vi "Motr_Ref_Num.vi"() -> (0 "Motor":T1)   [LabVIEW 2015]
uses:
  Motor_Type_Def.ctl
  <vilib>/Rock Robotics/WPI/RobotDrive/WPI_RobotDriveDevRef.ctl
  <vilib>/Rock Robotics/WPI/MotorControl/WPI_MotorControlDeviceRef.ctl
  <vilib>/Rock Robotics/WPI/MotorControl/WPI_MotorControlType.ctl
  <vilib>/Rock Robotics/SystemInterfaces/DIO/FPGA_DIOPWMChannel.ctl
  <vilib>/Rock Robotics/WPI/PWM/WPI_PWMDeadband.ctl
  <vilib>/Rock Robotics/WPI/CAN/Jaguar/SubVIs/WPI_CANJaguar_ControlMode.ctl
  <vilib>/Rock Robotics/WPI/CAN/TalonSRX/WPI_CANTalonSRX_APIControlMode.ctl
  <vilib>/Rock Robotics/WPI/Utilities/WPI_GetSetVariantRefNum.vi
panel:
  # "Made by Matt Carr on 1/30/2016"
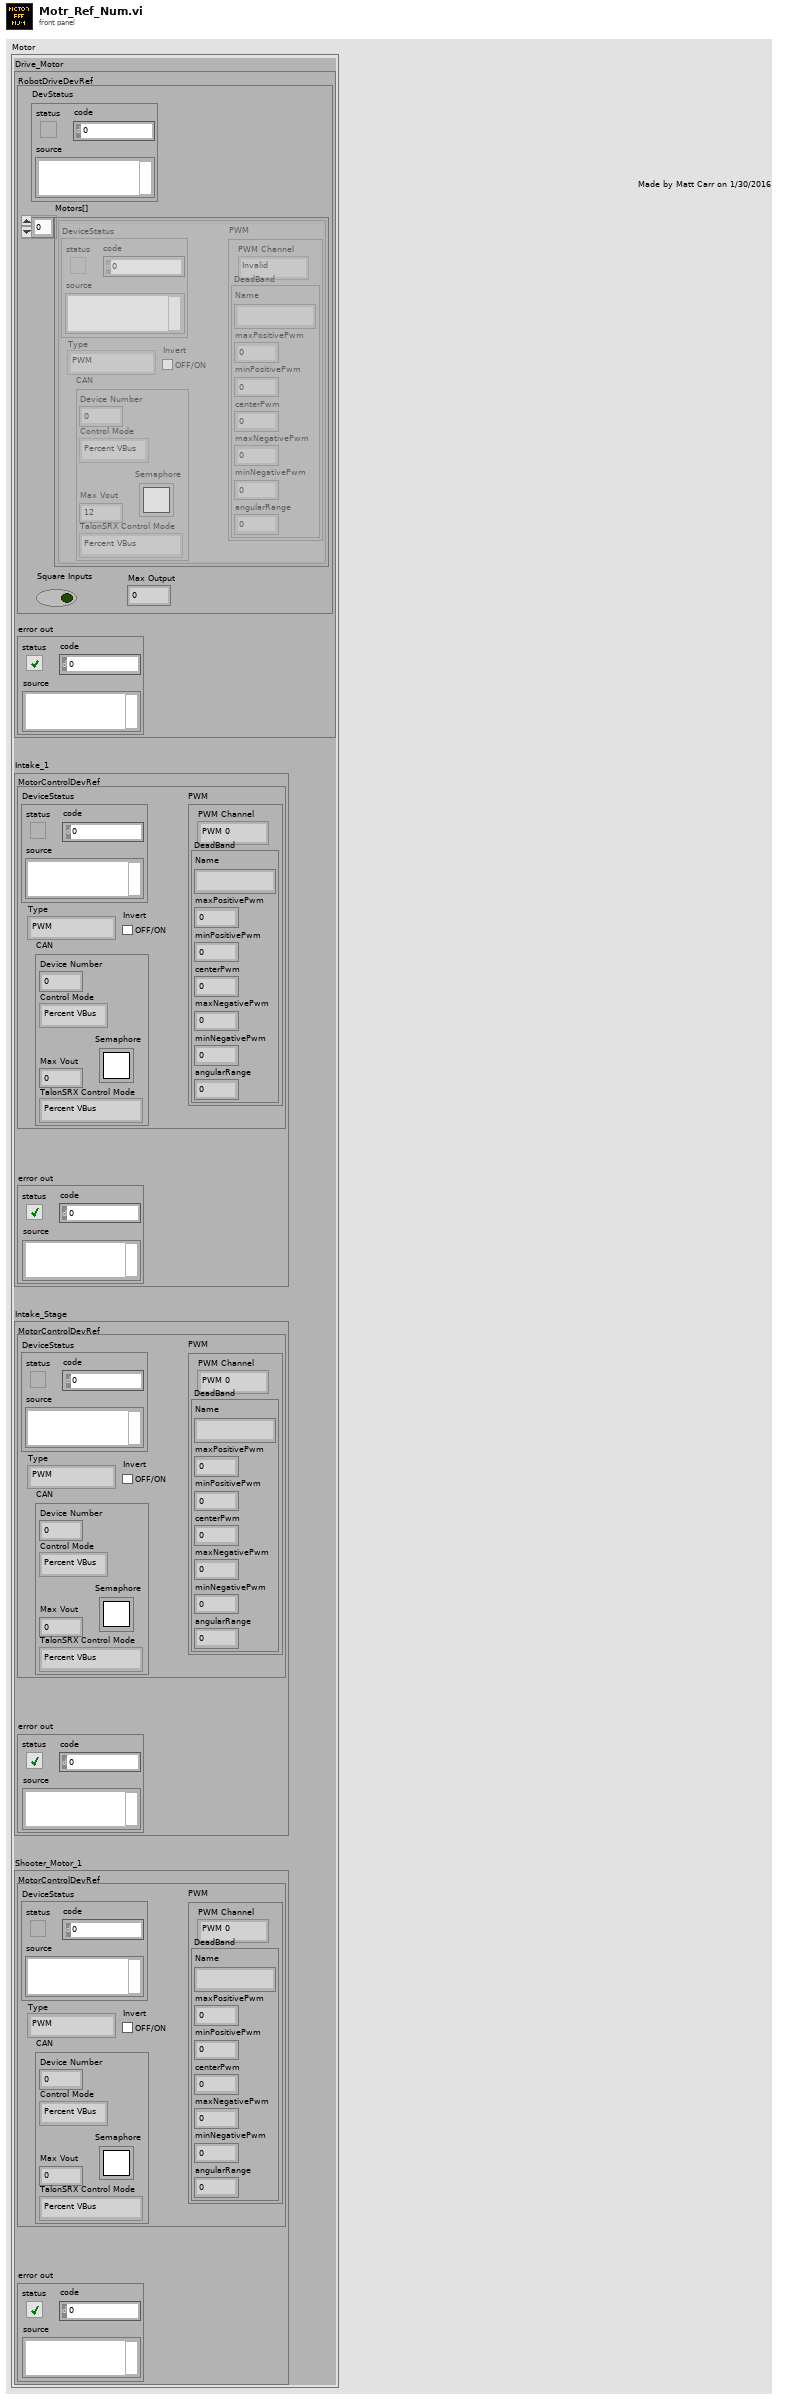
[diagram p1: front panel]
types:
  T1 = typedef "Motor_Type_Def.ctl" = cluster{"Drive_Motor":cluster{"RobotDriveDevRef":T2, "error out":errorcluster}, "Intake_1":cluster{"MotorControlDevRef":T3, "error out":errorcluster}, "Intake_Stage":cluster{"MotorControlDevRef":T3, "error out":errorcluster}, "Shooter_Motor_1":cluster{"MotorControlDevRef":T3, "error out":errorcluster}}
  T2 = typedef "WPI_RobotDriveDevRef.ctl" = cluster{"DevStatus":errorcluster, "Motors[]":T3[], "Square Inputs":bool, "Max Output":dbl}
  T3 = typedef "WPI_MotorControlDeviceRef.ctl" = cluster{"DeviceStatus":errorcluster, "Type":T4, "PWM":cluster{"PWM Channel":T5, "DeadBand":T6}, "CAN":cluster{"Device Number":u8, "Control Mode":T7, "Semaphore":T8, "Max Vout":dbl, "TalonSRX Control Mode":T9}, "Invert":bool}
  T4 = typedef "WPI_MotorControlType.ctl" = enum16{"PWM", "CAN", "CANTalonSRX"}
  T5 = typedef "FPGA_DIOPWMChannel.ctl" = enum8{"PWM 0", "PWM 1", "PWM 2", "PWM 3", "PWM 4", "PWM 5", "PWM 6", "PWM 7", "PWM 8", "PWM 9", "PWM MXP 0", "PWM MXP 1", "PWM MXP 2", "PWM MXP 3", "PWM MXP 4", "PWM MXP 5", "PWM MXP 6", "PWM MXP 7", "PWM MXP 8", "PWM MXP 9", "Invalid"}
  T6 = typedef "WPI_PWMDeadband.ctl" = cluster{"Name":string, "maxPositivePwm":i32, "minPositivePwm":i32, "centerPwm":i32, "maxNegativePwm":i32, "minNegativePwm":i32, "angularRange":u16}
  T7 = typedef "WPI_CANJaguar_ControlMode.ctl" = enum8{"Percent VBus", "Current", "Speed", "Position", "Voltage"}
  T8 = typedef "Semaphore RefNum" = refnum<k1>
  T9 = typedef "WPI_CANTalonSRX_APIControlMode.ctl" = enum8{"Percent VBus", "Speed", "Position", "Slave", "Unchanged / Invalid", "Voltage Compensation", "Current", "Motion Profile"}
  T10 = cluster{"MotorControlDevRef":T3, "error out":errorcluster}
  T11 = cluster{"RobotDriveDevRef":T2, "error out":errorcluster}
  T12 = cluster{"Drive_Motor":cluster{"RobotDriveDevRef":T2, "error out":errorcluster}, "Intake_1":cluster{"MotorControlDevRef":T3, "error out":errorcluster}, "Intake_Stage":cluster{"MotorControlDevRef":T3, "error out":errorcluster}, "Shooter_Motor_1":cluster{"MotorControlDevRef":T3, "error out":errorcluster}}
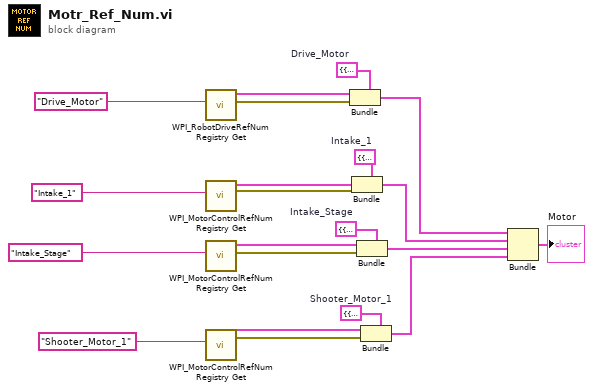
[diagram p0: block diagram]
diagram:
  w6 = T10 {"MotorControlDevRef"={"DeviceStatus"={"status"=FALSE, "code"=0, "source"=""}, "Type"=enum."PWM", "PWM"={"PWM Channel"=enum."PWM 0", "DeadBand"={"Name"="", "maxPositivePwm"=0, "minPositivePwm"=0, "centerPwm"=0, "maxNegativePwm"=0, "minNegativePwm"=0, "angularRange"=0}}, "CAN"={"Device Number"=0, "Control Mode"=enum."Percent VBus", "Semaphore"=refnum, "Max Vout"=0.0, "TalonSRX Control Mode"=enum."Percent VBus"}, "Invert"=FALSE}, "error out"={"status"=FALSE, "code"=0, "source"=""}}  # Shooter_Motor_1
  w8 = T10 {"MotorControlDevRef"={"DeviceStatus"={"status"=FALSE, "code"=0, "source"=""}, "Type"=enum."PWM", "PWM"={"PWM Channel"=enum."PWM 0", "DeadBand"={"Name"="", "maxPositivePwm"=0, "minPositivePwm"=0, "centerPwm"=0, "maxNegativePwm"=0, "minNegativePwm"=0, "angularRange"=0}}, "CAN"={"Device Number"=0, "Control Mode"=enum."Percent VBus", "Semaphore"=refnum, "Max Vout"=0.0, "TalonSRX Control Mode"=enum."Percent VBus"}, "Invert"=FALSE}, "error out"={"status"=FALSE, "code"=0, "source"=""}}  # Intake_Stage
  w9 = T10 {"MotorControlDevRef"={"DeviceStatus"={"status"=FALSE, "code"=0, "source"=""}, "Type"=enum."PWM", "PWM"={"PWM Channel"=enum."PWM 0", "DeadBand"={"Name"="", "maxPositivePwm"=0, "minPositivePwm"=0, "centerPwm"=0, "maxNegativePwm"=0, "minNegativePwm"=0, "angularRange"=0}}, "CAN"={"Device Number"=0, "Control Mode"=enum."Percent VBus", "Semaphore"=refnum, "Max Vout"=0.0, "TalonSRX Control Mode"=enum."Percent VBus"}, "Invert"=FALSE}, "error out"={"status"=FALSE, "code"=0, "source"=""}}  # Intake_1
  w11 = T11 {"RobotDriveDevRef"={"DevStatus"={"status"=FALSE, "code"=0, "source"=""}, "Motors[]"=[], "Square Inputs"=FALSE, "Max Output"=0.0}, "error out"={"status"=FALSE, "code"=0, "source"=""}}  # Drive_Motor
  n1 = call <vilib>:"WPI_RobotDriveRefNum Registry Get.vi"("refnum name"="Drive_Motor") -> ("error out"=w15:errorcluster, "RobotDriveDevRef"=w7:T2)  [unwired: 9 in]
  n2 = call <vilib>:"WPI_MotorControlRefNum Registry Get.vi"("refnum name"="Intake_1") -> ("error out"=w2:errorcluster, "MotorControlDevRef"=w10:T3)  [unwired: 9 in]
  n3 = call <vilib>:"WPI_MotorControlRefNum Registry Get.vi"("refnum name"="Intake_Stage") -> ("error out"=w19:errorcluster, "MotorControlDevRef"=w18:T3)  [unwired: 9 in]
  n4 = call <vilib>:"WPI_MotorControlRefNum Registry Get.vi"("refnum name"="Shooter_Motor_1") -> ("error out"=w3:errorcluster, "MotorControlDevRef"=w16:T3)  [unwired: 9 in]
  n5 = Bundle(cluster=w11, "RobotDriveDevRef"=w7, "error out"=w15) -> (w1:T11)
  n6 = Bundle(cluster=w9, "MotorControlDevRef"=w10, "error out"=w2) -> (w14:T10)
  n7 = Bundle(cluster=w8, "MotorControlDevRef"=w18, "error out"=w19) -> (w13:T10)
  n8 = Bundle(cluster=w6, "MotorControlDevRef"=w16, "error out"=w3) -> (w12:T10)
  n9 = Bundle("Drive_Motor"=w1, "Intake_1"=w14, "Intake_Stage"=w13, "Shooter_Motor_1"=w12) -> (→"Motor":T12)  [unwired: 1 in]
